vi "Stop Button.vi"   [LabVIEW 2019]
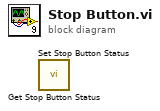
[diagram p0: block diagram]
diagram:
  n1 = call "Get Stop Button Status.vi"() -> ()  [unwired: 10 in, 2 out]
  n2 = call "Set Stop Button Status.vi"() -> ()  [unwired: 11 in, 1 out]
